vi "ExMoveSpectroMult.vi"() -> ()   [LabVIEW 2010]
panel:
  in  "Spectrometer Number":i16=1 min=1 max=64 step=1
  out "Current Wavelength":string
  in  "Increment Wavelength":dbl=50.0 format="%.2f"
  in  "End Wavelength":dbl=700.0 format="%.2f"
  in  "Start Wavelength":dbl format="%.2f"
  in  "Grating Speed":dbl=2000.0 min=1.0 step=1.0 format="%.2f"
  in  "Grating number":i16=1 min=1 max=100 step=1
  out "error out":errorcluster
  in  "error in (no error)":errorcluster
  # "ExMoveSpectroMult.vi\n(Normal Spectrograph via USB/COM port)\nThis VI is a simple example of how to setup and move a spectrograph in increments over a wavelength range."
  # "NOTES:\nA properly configured spectometer .ini must be present in the LabVIEW folder for spectrograph operation.\n\nConsult the Toolkit documentation for more information on how to configure this file."
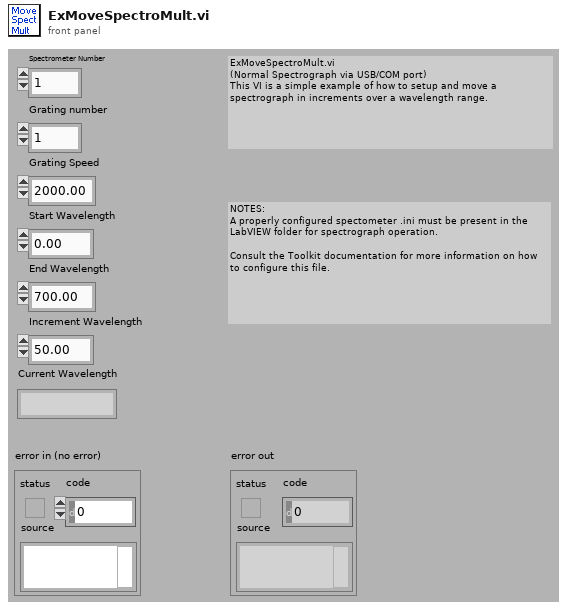
[diagram p1: front panel]
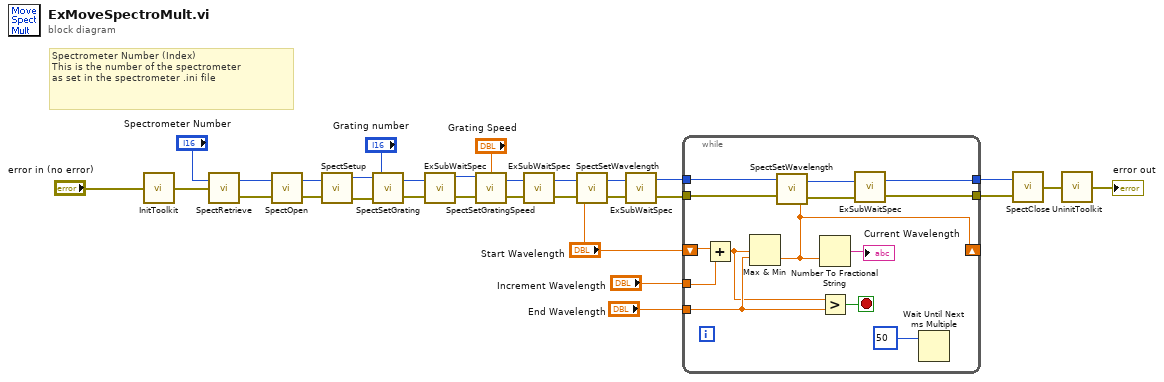
[diagram p0: block diagram]
diagram:
  # "Spectrometer Number (Index)\nThis is the number of the spectrometer\nas set in the spectrometer .ini file"
  n1 = call <userlib>:"InitToolkit.vi"("error in"="error in (no error)") -> ("error out"=w6:errorcluster)
  n2 = call <userlib>:"SpectRetrieve.vi"("error in"=w6, "Index"="Spectrometer Number") -> ("error out"=w5:errorcluster, "Device ID"=w3:u32)
  n3 = call <userlib>:"SpectOpen.vi"("error in"=w5, "Spectrometer ID"=w3) -> ("error out"=w10:errorcluster, "Spectrometer Handle"=w12:u32)  [unwired: 1 in]
  n4 = call <userlib>:"SpectSetup.vi"("error in"=w10, "Spectrometer Handle"=w12) -> ("error out"=w9:errorcluster, "Spectrometer Handle"=w11:u32)
  n5 = call <userlib>:"SpectSetGrating.vi"("error in"=w9, "Grating Number"="Grating number", "Sepctrometer Handle"=w11) -> ("error out"=w18:errorcluster, "Spectrometer Handle"=w17:u32)
  n6 = call "ExSubWaitSpec.vi"("error in (no error)"=w18, "Spectrometer Handle"=w17) -> ("error out"=w16:errorcluster, "Spectrometer handle"=w15:u32)
  n7 = call <userlib>:"SpectSetGratingSpeed.vi"("error in"=w16, "Grating Speed"="Grating Speed", "Spectrometer Handle"=w15) -> ("error out"=w13:errorcluster, "Spectrometer Handle"=w14:u32)
  n8 = call "ExSubWaitSpec.vi"("error in (no error)"=w13, "Spectrometer Handle"=w14) -> ("error out"=w1:errorcluster, "Spectrometer handle"=w2:u32)
  n9 = call <userlib>:"SpectSetWavelength.vi"("error in"=w1, "Wavelength"="Start Wavelength", "Spectrometer Handle"=w2) -> ("error out"=w30:errorcluster, "Spectrumeter Handle"=w29:u32)
  n10 = call "ExSubWaitSpec.vi"("error in (no error)"=w30, "Spectrometer Handle"=w29) -> ("error out"=w22:errorcluster, "Spectrometer handle"=w28:u32)
  n11 = while {
    tunnel: w28 -> [w35]
    tunnel: "Increment Wavelength" -> [w42]
    tunnel: "End Wavelength" -> [w34]
    shift-right: [w32] -> _
    shift-left: "Start Wavelength" -> [w43]
    tunnel: [w39] -> w24
    tunnel: [w36] -> w23
    tunnel: w22 -> [w38]
    stop <- w33 stop-if-true
    n12 = Add(x=w43, y=w42) -> (x+y=w31:dbl)
    n13 = Max & Min(x=w31, y=w34) -> (min(x,y)=w32:dbl)  [unwired: 1 out]
    n14 = call <userlib>:"SpectSetWavelength.vi"("error in"=w38, "Wavelength"=w32, "Spectrometer Handle"=w35) -> ("error out"=w37:errorcluster, "Spectrumeter Handle"=w40:u32)
    n15 = Number To Fractional String(number=w32) -> (F-format string=→"Current Wavelength":string)  [unwired: 3 in]
    n16 = Greater?(x=w31, y=w34) -> (0:w33:bool)
    n17 = call "ExSubWaitSpec.vi"("error in (no error)"=w37, "Spectrometer Handle"=w40) -> ("error out"=w36:errorcluster, "Spectrometer handle"=w39:u32)
    n18 = Wait Until Next ms Multiple(millisecond multiple=50) -> ()  [unwired: 1 out]
  }
  n19 = call <userlib>:"SpectClose.vi"("error in"=w23, "Spectrometer Handle"=w24) -> ("error out"=w20:errorcluster)
  n20 = call <userlib>:"UninitToolkit.vi"("error in"=w20) -> ("error out"=→"error out":errorcluster)
